vi "ClusterToStruct.vi"(7 "String Taget Alignment (1)":i32=1, 8 "error in (no error)":errorcluster, 9 "byte order (1, host order checking)":T3(ring)=enum."native, host order", 10 "#pragma packing directive (0, default)":i32, 11 "LV Cluster":variant) -> (0 "error out":errorcluster, 1 "byte order Used":T3(ring)=enum."native, host order", 2 "Element and Padding Info":T1, 3 "Cluster Data as Byte Array Out":u8[](array[numeric]), 5 "Struct Size":i32)   [LabVIEW 2020]
doc: "Pass any Cluster to the function (it will auto-cast to a variant), and return the cluster data as a byte array which can be used by a CLFN to a DLL expecting a C Sturct.\n\nIn the CLFN parameter use:\nType = Array,\nData Type = Unsigned 8-bit Integer,\nArray Format = Array Data Pointer,\nMinimum Size = None.\n\nUse this function to format a LabVIEW cluster into a universal byte array that replicates the correct packing and endian-ness of a C Struct that a subsequently executed DLL function call may be expecting. \n\nDepending on the DLL, the data elements in a Struct may be represented in memory-space with specific \"endian-ness\" as well as specific \"padding\" between certain elements of the Struct. LabVIEW Clusters and most C Struct are similar in that data element B always follow element A <b> however, </b> LV assumes 1-byte packing (no padding) while the default C packing is NOT 1-byte and moreover, may be explicitly defined by the compiler directive \"#pragma pack\".\n\n\"Endian-ness\" refers to how data element bytes are ordered in memory. Most (all?) Windows machines are little endian. This function includes the ability to check host endian-ness."
uses:
  TypeDefs/ctl_ElementAndPaddingInfo.ctl
  TypeDefs/ctl_DataElementInfo.ctl
panel:
  # "### BSD License (http://www.opensource.org/licenses/bsd-license.php) Begin ###\n \nCopyright (c) 2014 Jeffrey Holt <jolt.holt@gmail.com>\n\nAll rights reserved.\n\nRedistribution and use in source and binary forms, with or without modification, are permitted provided that the following conditions are met:\n\n    * Redistributions of source code must retain the above copyright notice\n\nTHIS SOFTWARE IS PROVIDED BY THE COPYRIGHT HOLDERS AND CONTRIBUTORS \"AS IS\" AND ANY EXPRESS OR IMPLIED WARRANTIES, \nINCLUDING, BUT NOT LIMITED TO, THE IMPLIED WARRANTIES OF MERCHANTABILITY AND FITNESS FOR A PARTICULAR PURPOSE ARE \nDISCLAIMED. IN NO EVENT SHALL THE COPYRIGHT OWNER OR CONTRIBUTORS BE LIABLE FOR ANY DIRECT, INDIRECT, INCIDENTAL,\n SPECIAL, EXEMPLARY, OR CONSEQUENTIAL DAMAGES (INCLUDING, BUT NOT LIMITED TO, PROCUREMENT OF SUBSTITUTE GOODS OR \nSERVICES; LOSS OF USE, DATA, OR PROFITS; OR BUSINESS INTERRUPTION) HOWEVER CAUSED AND ON ANY THEORY OF LIABILITY, \nWHETHER IN CONTRACT, STRICT LIABILITY, OR TORT (INCLUDING NEGLIGENCE OR OTHERWISE) ARISING IN ANY WAY OUT OF THE USE \nOF THIS SOFTWARE, EVEN IF ADVISED OF THE POSSIBILITY OF SUCH DAMAGE.\n\n### BSD License End ###"
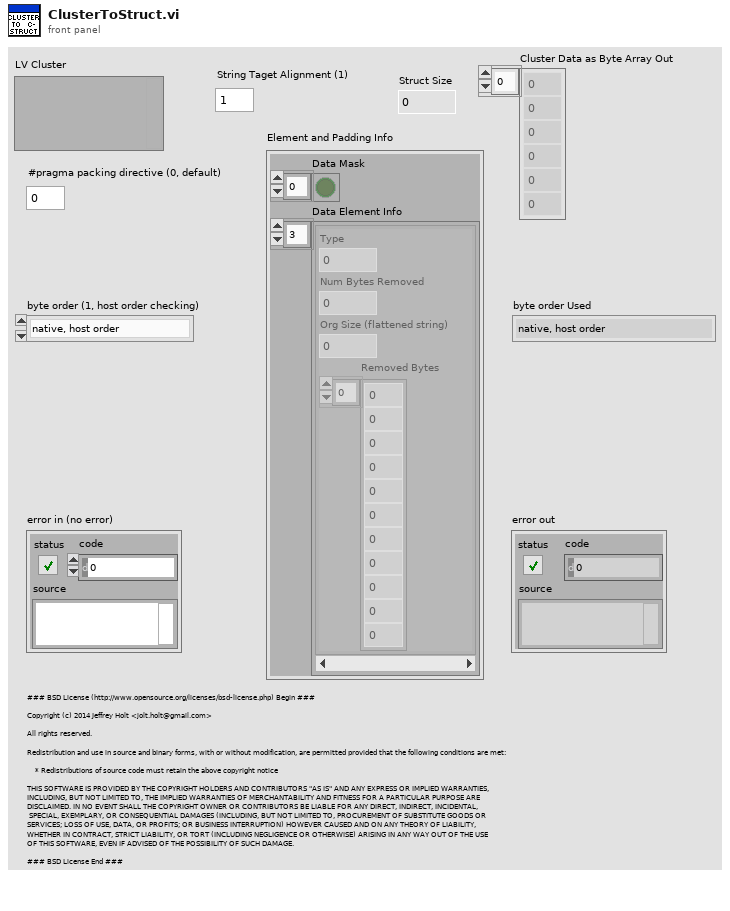
[diagram p1: front panel]
types:
  T1 = typedef "ctl_ElementAndPaddingInfo.ctl" = cluster{"Data Mask":bool[], "Data Element Info":T2[]}
  T2 = typedef "ctl_DataElementInfo.ctl" = cluster{"Type":u16, "Num Bytes Removed":u16, "Org Size (flattened string)":i32, "Removed Bytes":u8[]}
  T3 = enum16{"big-endian, network order", "native, host order", "little-endian"}
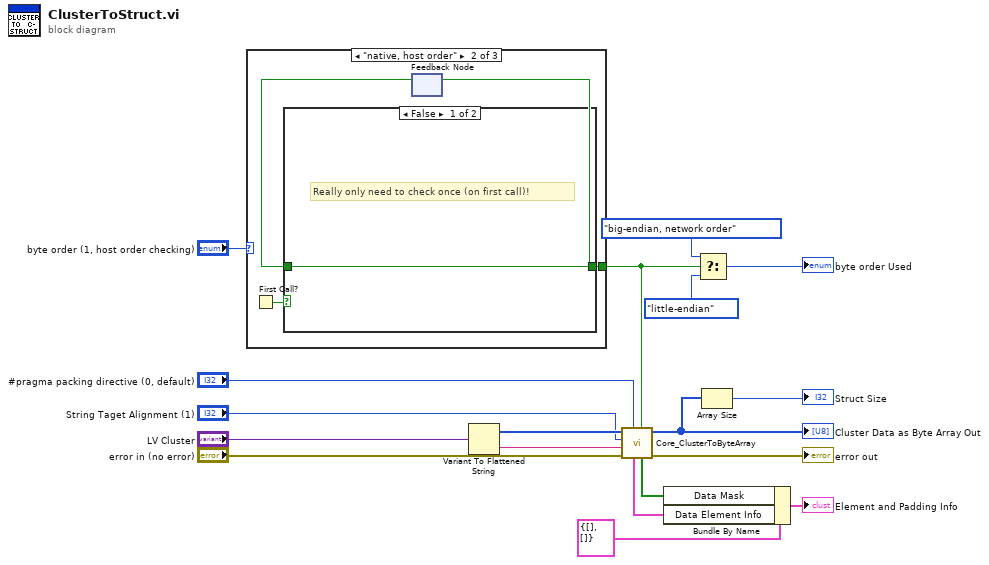
[diagram p0: block diagram]
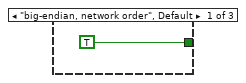
[diagram p2: hidden frame]
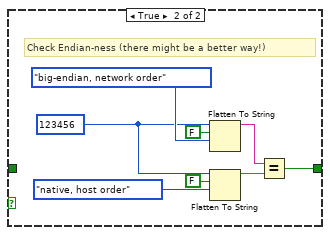
[diagram p3: hidden frame]
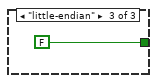
[diagram p4: hidden frame]
diagram:
  n1 = case shown="\"native, host order\"" "byte order (1, host order checking)" {
    tunnel: [TRUE w22 FALSE] -> w8
    frame "big-endian, network order", Default {
    }
    frame "native, host order" {
      n2 = First Call?() -> (First Call?: T/F=w21:bool)
      n3 = feedback #1() -> (w20:bool)  [unwired: 1 in]
      n4 = case shown="False" w21 {
        tunnel: [w23 w24] -> w22
        tunnel: w20 -> [w23 _]
        frame False {
          # "Really only need to check once (on first call)!"
        }
        frame True {
          w25 = 123456
          # "Check Endian-ness (there might be a better way!)"
          n5 = Flatten To String(anything=w25, prepend array or string size? (T)=FALSE, byte order (0:big-endian, network order)=T3."big-endian, network order") -> (data string=w27:string)  [unwired: 1 in, 2 out]
          n6 = Flatten To String(anything=w25, prepend array or string size? (T)=FALSE, byte order (0:big-endian, network order)=T3."native, host order") -> (data string=w26:string)  [unwired: 1 in, 2 out]
          n7 = Equal?(x=w27, y=w26) -> (x = y?=w24:bool)
        }
      }
      n8 = feedback-in #1(w22) -> ()
    }
    frame "little-endian" {
    }
  }
  n9 = Variant To Flattened String(Variant="LV Cluster") -> (data string=w12:string, 1:w11:i16[])
  n10 = call "Core_ClusterToByteArray.vi"("Endian-ness (T, Big)"=w8, "#pragma directive (0, default)"="#pragma packing directive (0, default)", "error in (no error)"="error in (no error)", "data string (big endian)"=w12, "String Taget Alignment (1)"="String Taget Alignment (1)", "type string"=w11) -> ("error out"=→"error out":errorcluster, "Cluster Data as Byte Array Out"=w15:u8[], "Data Mask"=w5:bool[], "Base Data Element Info"=w4:T2[])  [unwired: 2 out]
  "Cluster Data as Byte Array Out" <- w15
  n11 = Bundle By Name(cluster=T1 {"Data Mask"=[], "Data Element Info"=[]} ("Element and Padding Info"), "Data Mask"=w5, "Data Element Info"=w4) -> (→"Element and Padding Info":T1)
  n12 = Select(t=T3."big-endian, network order" ("byte order (1, host order checking)"), s=w8, f=T3."little-endian" ("byte order (1, host order checking)")) -> (s? t:f=→"byte order Used":T3)
  n13 = Array Size(array=w15) -> (size(s)=→"Struct Size":i32)
